vi "Control Mode.vi"(8 "error in (no error)":errorcluster, 11 "BoardHandle":T1) -> (0 "error out":errorcluster, 1 "Remote enable?":bool, 2 "Control mode":string, 3 "BoardHandle out":T1)   [LabVIEW 2019, in "CAEN PSM.lvlib"]
doc: "This function allows to know the control mode setting."
uses:
  Users/pcmmegas02/Downloads/CAEN_PSM-InstrumentDriver-1.0.2/CAEN PSM/CAEN PSM.lvlib
  Users/pcmmegas02/Downloads/CAEN_PSM-InstrumentDriver-1.0.2/CAEN PSM/Private/BoardHandle.ctl
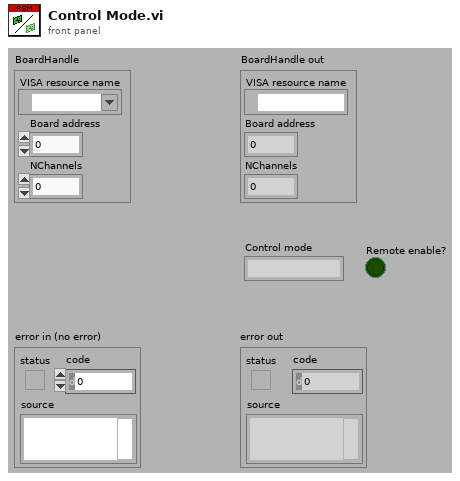
[diagram p1: front panel]
types:
  T1 = typedef "CAEN PSM.lvlib/BoardHandle.ctl" = cluster{"VISA resource name":refnum<visa-resource-name>, "Board address":u8, "NChannels":u8}
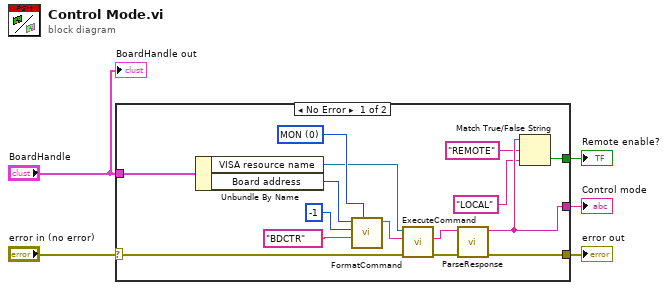
[diagram p0: block diagram]
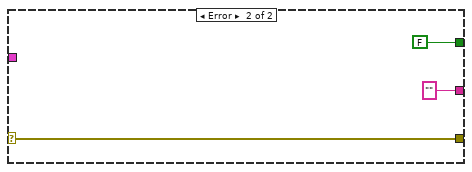
[diagram p2: hidden frame]
diagram:
  n1 = case shown="No Error" "error in (no error)" {
    selector: "error in (no error)" -> [w12 w23]
    tunnel: [w15 w23] -> w4
    tunnel: "BoardHandle" -> [w13 _]
    tunnel: [w9 "" ("val")] -> w2
    tunnel: [w6 FALSE ("selection")] -> w1
    frame No Error {
      w19 = u8 0 items=["MON", "SET"] ("CMD")
      n2 = Unbundle By Name(w13) -> ("VISA resource name"=w18:refnum<visa-resource-name>, "Board address"=w20:u8)
      n3 = call "FormatCommand.vi"("CMD (MON)"=w19, "PAR"="BDCTR", "CH"=i8 -1, "BD (0)"=w20) -> ("cmd"=w17:string)  [unwired: 7 in]
      n4 = call "ExecuteCommand.vi"("error in (no error)"=w12, "Command"=w17, "VISA resource name"=w18) -> ("error out"=w16:errorcluster, "Response"=w14:string)  [unwired: 6 in, 1 out]
      n5 = call "ParseResponse.vi"("error in (no error)"=w16, "Response"=w14) -> ("error out"=w15:errorcluster, "val"=w9:string)  [unwired: 6 in, 2 out]
      n6 = Match True/False String(2:"LOCAL" ("false string"), 3:"REMOTE" ("true string"), 4:w9) -> (0:w6:bool)  [unwired: 1 out]
    }
    frame Error {
    }
  }
  "error out" <- w4
  "Control mode" <- w2
  "Remote enable?" <- w1
  "BoardHandle out" <- "BoardHandle"
